vi "JDT.vi"(0 "System no.":i32=1 min=1 max=4 step=1, 1 "Joystick ID":i32[](array[numeric]), 2 "Joystick axis":i32[](array[numeric]), 3 "Lookup table type":i32[](array[numeric]), 5 "error in":errorcluster) -> (14 "Controller error":bool, 19 "error out":errorcluster)   [LabVIEW 2020]
doc: "Sets default lookup table for joysticks connected to the controller, waits 100 ms and queries ERR?. \nController error is TRUE if selected system reports error code ? 0. Settings will not influence Joystick_Operation_Sample_Program.vi which works with a joystick connected to the host computer.\n\nC-867, E-709, E-861, Mercury_GCS: The following default lookup tables are provided:\n1 = linear\n2 = parabolic\n\nE-709: Only supported if E-709 is used inside C-867K012/K013.\n\nE-870: The following default lookup tables are provided:\n1 = linear\n2 = parabolic\n5 = linear invert\n6 = parabolic invert\n\nMercury: The following default lookup tables are provided:\n1 = linear\n3 = cubic"
panel:
  # "Sets default lookup table for joysticks connected to the controller."
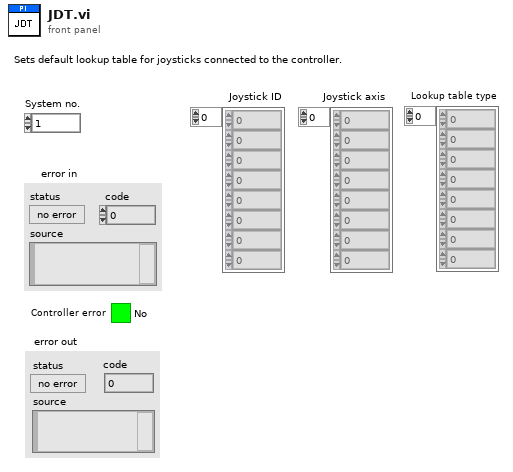
[diagram p1: front panel]
types:
  T1 = enum16{"Disable error check", "Force error check", "Use global settings"}
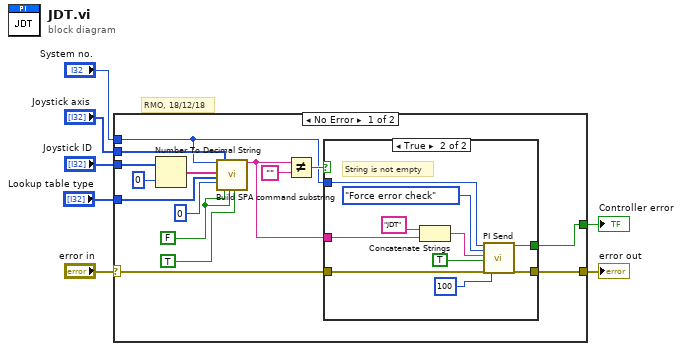
[diagram p0: block diagram]
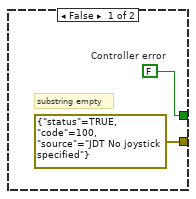
[diagram p2: hidden frame]
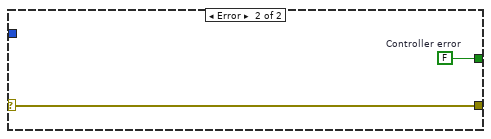
[diagram p3: hidden frame]
diagram:
  # "RMO, 18/12/18"
  n1 = case shown="No Error" "error in" {
    selector: "error in" -> [w9 w36]
    tunnel: [w22 w36] -> w7
    tunnel: "Lookup table type" -> [w19 _]
    tunnel: "System no." -> [w16 _]
    tunnel: "Joystick ID" -> [w14 _]
    tunnel: "Joystick axis" -> [w18 _]
    tunnel: [w8 w35] -> w1
    frame No Error {
      w12 = FALSE ("Parameter no. format \n(Decimal: FALSE)")
      n2 = Number To Decimal String(number=w14, width (-)=i16 0) -> (decimal integer string=w13:string[])
      n3 = call "Build SPA command substring.vi"("System no."=w16, "Axes to set"=w13, "Parameter values"=w19, "No. of digits"=i16 0, "Parameter number"=w18, "Parameter no. format \n(Decimal: FALSE)"=w12, "Parameter format \n(Num.: FALSE)"=w12, "With space?"=TRUE) -> ("SPA command substring"=w20:string)  [unwired: 2 in, 9 out]
      n4 = Not Equal?(x=w20, y="") -> (x != y?=w17:bool)
      n5 = case shown="True" w17 {
        tunnel: w20 -> [_ w33]
        tunnel: [errorcluster {"status"=TRUE, "code"=100, "source"="JDT No joystick specified"} ("error out") w25] -> w22
        tunnel: w9 -> [_ w30]
        tunnel: w16 -> [_ w29]
        tunnel: [w23 w26] -> w8
        frame False {
          w23 = FALSE  # Controller error
          # "substring empty"
        }
        frame True {
          # "String is not empty"
          n6 = Concatenate Strings("JDT", w33) -> (w31:string)
          n7 = call "PI Send.vi"("System no."=w29, "Error check settings"=T1."Force error check", "String to send"=w31, "Attach termination char.?"=TRUE ("Attach Linefeed?"), "error in"=w30, "Delay before error check (ms)"=u32 100 ("milliseconds to wait")) -> ("Controller error"=w26:bool, "error out"=w25:errorcluster)  [unwired: 12 out]
        }
      }
    }
    frame Error {
      w35 = FALSE  # Controller error
    }
  }
  "error out" <- w7
  "Controller error" <- w1
